vi "SUB_SORT_2D_ARRAY.vi"(8 "Index sort by":i32, 11 "array":string[][](array[string])) -> (3 "Sorted array":string[][](array[string]))   [LabVIEW 2015]
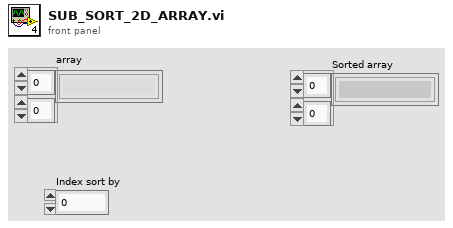
[diagram p1: front panel]
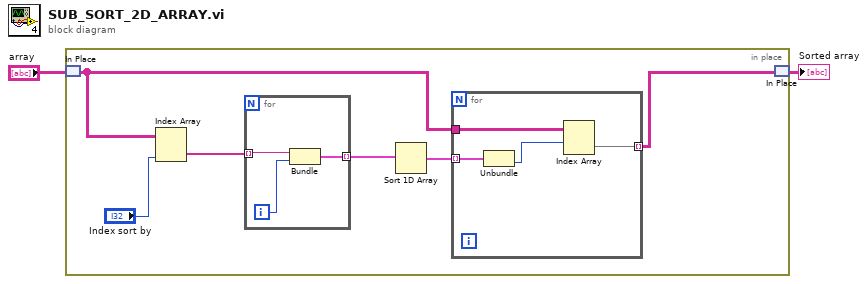
[diagram p0: block diagram]
diagram:
  n1 = in-place {
    n2 = in-place-match #1("array") -> (w4:string[][])
    n3 = Index Array(array=w4, index (col)="Index sort by") -> (element=w7:string[])  [unwired: 1 in]
    n4 = for {
      tunnel: w7 -> [w14] mode=indexing
      tunnel: [w13] -> w6 mode=indexing
      i -> [w15]
      n5 = Bundle("문자열"=w14, w15) -> (w13:cluster{"문자열":string, i32})  [unwired: 1 in]
    }
    n6 = Sort 1D Array(array=w6) -> (sorted array=w5:cluster{"문자열":string, i32}[])
    n7 = for {
      tunnel: w5 -> [w12] mode=indexing
      tunnel: w4 -> [w11]
      tunnel: [w9] -> w3 mode=indexing
      n8 = Unbundle(w12) -> (w10:i32)  [unwired: 1 out]
      n9 = Index Array(array=w11, index (row)=w10) -> (element=w9:string[])  [unwired: 1 in]
    }
    n10 = in-place-match #1(w3) -> (→"Sorted array":string[][])
  }
